vi "Create Plugin Template.vi"(0 "project path":path, 5 "description":string, 11 "error in":errorcluster) -> (15 "error out":errorcluster)   [LabVIEW 2021, in "Converter.lvlib"]
uses:
  Converter.lvlib
  Measurement Plugin Generator/_MeasurementService Utility/MeasurementService Editor.lvlib
  Converter Reusables/Converter Reusables.lvlib
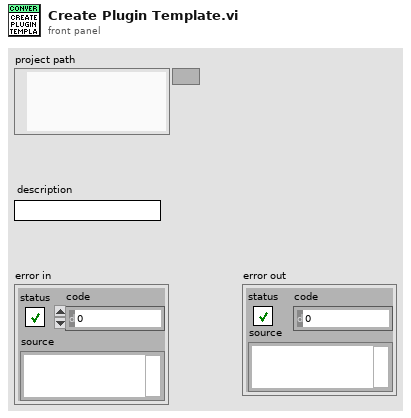
[diagram p1: front panel]
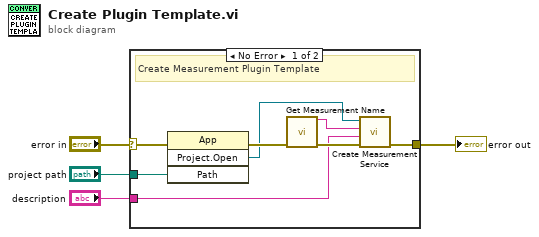
[diagram p0: block diagram]
diagram:
  n1 = case shown="No Error" "error in" {
    selector: "error in" -> [w10 w13]
    tunnel: "project path" -> [w9 _]
    tunnel: [w11 w13] -> w2
    tunnel: "description" -> [w5 _]
    frame No Error {
      # "Create Measurement Plugin Template"
      n2 = invoke class="App" method="Project.Open"(error in=w10, "Path"=w9) -> (error out=w8:errorcluster, "Project:Open"=w6:refnum<vi>)  [unwired: 2 in, 2 out]
      n3 = call "Get Measurement Name.vi"("error in"=w8) -> ("name out"=w7:string, "error out"=w12:errorcluster)  [unwired: 13 in]
      n4 = call "Create Measurement Service.vi"("error in"=w12, "measurement plug-in description"=w5, "measurement plug-in name"=w7, "project ref"=w6) -> ("error out"=w11:errorcluster)  [unwired: 7 in]
    }
    frame Error {
    }
  }
  "error out" <- w2
